vi "AutoRotate.vi"(1 "Speed":dbl=1.0 format="%#_13g", 2 "Degrees":dbl=90.0 format="%#_13g", 3 "Clockwise?":bool) -> (0 "Distance (ft)":dbl)   [LabVIEW 2014]
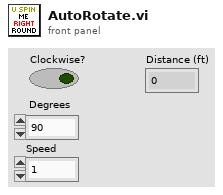
[diagram p1: front panel]
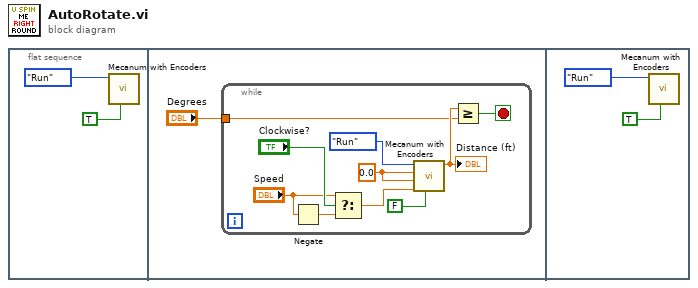
[diagram p0: block diagram]
diagram:
  n1 = flat-sequence {
    frame #0 {
      n2 = call "Mecanum with Encoders.vi"("Reset"=TRUE, "Mode"=enum8{"Start", "Run", "Finish"}."Run") -> ()  [unwired: 8 in, 1 out]
    }
    frame #1 {
      n3 = while {
        tunnel: "Degrees" -> [w11]
        stop <- w10 stop-if-true
        w4 = 0.0 ("Strafe")
        n4 = Negate(x="Speed") -> (-x=w6:dbl)
        n5 = Select(t="Speed", s="Clockwise?", f=w6) -> (s? t:f=w5:dbl)
        n6 = call "Mecanum with Encoders.vi"("Reset"=FALSE, "Turn"=w5, "Forward/Backward"=w4, "Strafe"=w4, "Mode"=enum8{"Start", "Run", "Finish"}."Run") -> ("Distance (ft)"=w12:dbl)  [unwired: 5 in]
        "Distance (ft)" <- w12
        n7 = Greater Or Equal?(x=w12, y=w11) -> (x >= y?=w10:bool)
      }
    }
    frame #2 {
      n8 = call "Mecanum with Encoders.vi"("Reset"=TRUE, "Mode"=enum8{"Start", "Run", "Finish"}."Run") -> ()  [unwired: 8 in, 1 out]
    }
  }
